vi "Compile Driver Configuration.vi"(8 "error in (no error)":errorcluster, 11 "Device Ref in":T1 format="%.0x") -> (0 "error out":errorcluster, 2 "Driver Configuration":T2, 3 "Device Ref out":T1 format="%.0x")   [LabVIEW 2017, in "SLSC Switch System Explorer.lvlib"]
uses:
  SLSC Switch System Explorer.lvlib
  Shared/Driver Configuration.ctl
  <vilib>/NI Veristand/Custom Device API/Custom Device Item Ref.ctl
  Scripting/SLSC Switch Scripting.lvlib
  Shared/SLSC Switch Shared.lvlib
  <vilib>/NI Veristand/Custom Device API/Custom Device API.lvlib
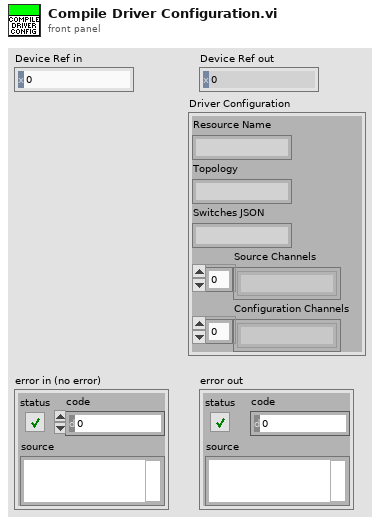
[diagram p1: front panel]
types:
  T1 = typedef "Custom Device API.lvlib/Custom Device Item Ref.ctl" = u64
  T2 = typedef "SLSC Switch Shared.lvlib/Driver Configuration.ctl" = cluster{"Resource Name":string, "Topology":string, "Switches JSON":string, "Source Channels":string[], "Configuration Channels":string[]}
  T3 = typedef "SLSC Switch Scripting.lvlib/SLSC Switch All Properties.ctl" = cluster{"Model":string, "Resource":string, "Topology":string, "Capabilities":string, "Description":string}
  T4 = typedef "SLSC Switch Shared.lvlib/Endpoint Configuration Cluster.ctl" = cluster{"Endpoint":string, "Configuration":T5}
  T5 = typedef "SLSC Switch Shared.lvlib/Endpoint Configuration Enum.ctl" = enum16{"Load", "Source", "Configuration"}
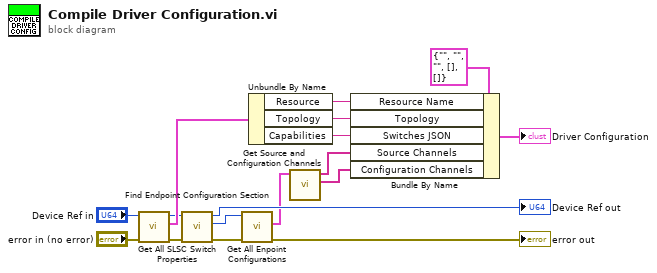
[diagram p0: block diagram]
diagram:
  n1 = call "Get All SLSC Switch Properties.vi"("error in (no error)"="error in (no error)", "SLSC Switch Custom Device Ref in"="Device Ref in") -> ("error out"=w8:errorcluster, "SLSC Switch All Properties"=w11:T3, "SLSC Switch Custom Device Ref out"=w7:T1)  [unwired: 7 in]
  n2 = call "Find Endpoint Configuration Section.vi"("error in (no error)"=w8, "SLSC Switch Custom Device Ref in"=w7) -> ("error out"=w6:errorcluster, "Endpoint Config Section Ref"=w5:T1, "SLSC Switch Custom Device Ref out"=→"Device Ref out":T1)  [unwired: 7 in]
  n3 = call "Get All Enpoint Configurations.vi"("error in (no error)"=w6, "Endpoint Configuration Section Ref in"=w5) -> ("error out"=→"error out":errorcluster, "All Endpoint Configurations"=w3:T4[])  [unwired: 7 in, 1 out]
  n4 = Unbundle By Name(w11) -> ("Resource"=w13:string, "Topology"=w14:string, "Capabilities"=w15:string)
  n5 = call "Get Source and Configuration Channels.vi"("All Endpoint Configurations"=w3) -> ("Configuration Channels"=w1:string[], "Source Channels"=w2:string[])  [unwired: 9 in]
  n6 = Bundle By Name(cluster=T2 {"Resource Name"="", "Topology"="", "Switches JSON"="", "Source Channels"=[], "Configuration Channels"=[]} ("Driver Configuration"), "Resource Name"=w13, "Topology"=w14, "Switches JSON"=w15, "Source Channels"=w2, "Configuration Channels"=w1) -> (→"Driver Configuration":T2)
